vi "udp-connectie.vi"() -> ()   [LabVIEW 2019]
panel:
  in  "port":u16
  in  "achteruit":bool
  in  "vooruit":bool
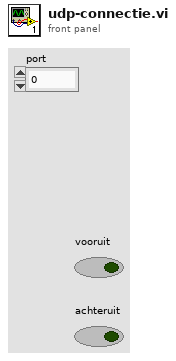
[diagram p1: front panel]
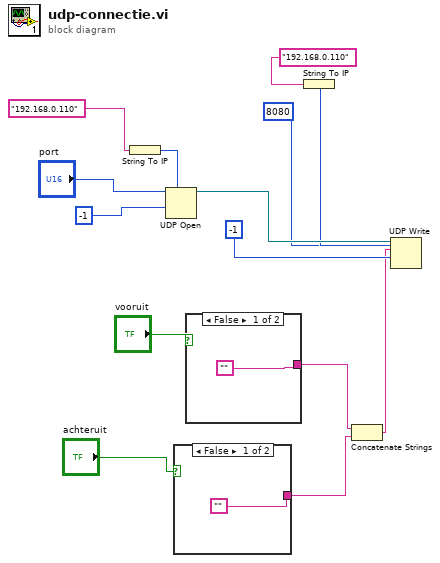
[diagram p0: block diagram]
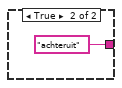
[diagram p2: hidden frame]
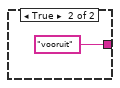
[diagram p3: hidden frame]
diagram:
  n1 = String To IP(1:"192.168.0.110") -> (0:w14:u32)
  n2 = UDP Open(7:w14, 9:-1 ("timeout ms (25000)"), 11:"port") -> (port=w11:refnum<k16>)  [unwired: 2 in, 2 out]
  n3 = case shown="False" "achteruit" {
    tunnel: ["" "achteruit"] -> w3
    frame False {
    }
    frame True {
    }
  }
  n4 = case shown="False" "vooruit" {
    tunnel: ["" "vooruit"] -> w4
    frame False {
    }
    frame True {
    }
  }
  n5 = String To IP(1:"192.168.0.110") -> (0:w10:u32)
  n6 = Concatenate Strings(w4, w3) -> (w2:string)
  n7 = UDP Write(address=w10, port or service name=8080, connection ID=w11, data in=w2, 9:-1 ("timeout ms (25000)")) -> ()  [unwired: 1 in, 2 out]
